vi "controllight.vi"() -> ()   [LabVIEW 2021]
uses:
  <vilib>/Instr/_visa.llb/VISA Configure Serial Port (Instr).vi
panel:
  in  "Reset":bool
  out "TIME":string
  out "Do sang":string
  out "qua toi":bool
  out "qua sang":bool
  out "do sang binh thuong":bool
  out "Waveform Chart":i32(graph)
  in  "write buffer":string
  in  "stop":bool
  out "read buffer":string
  in  "VISA resource name":refnum<visa-resource-name>
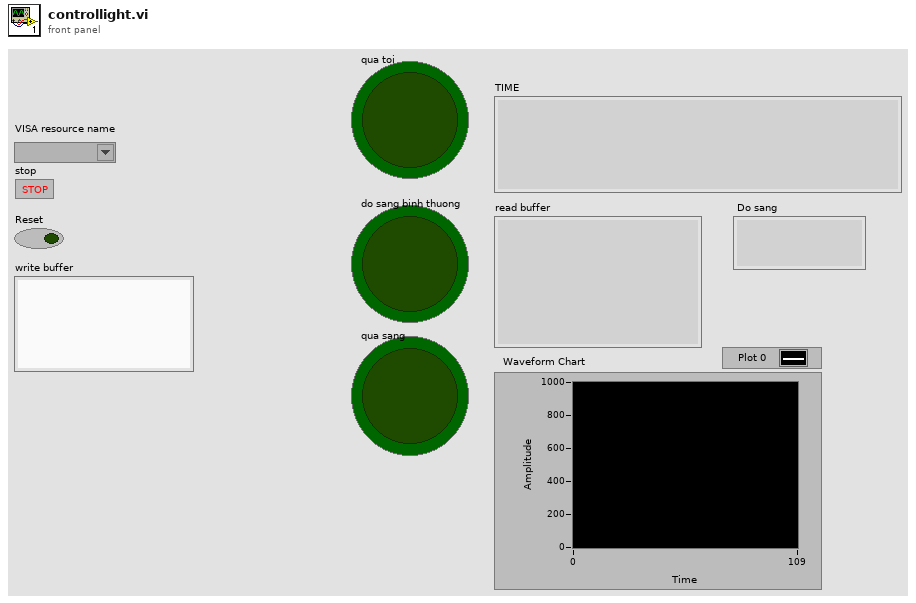
[diagram p1: front panel]
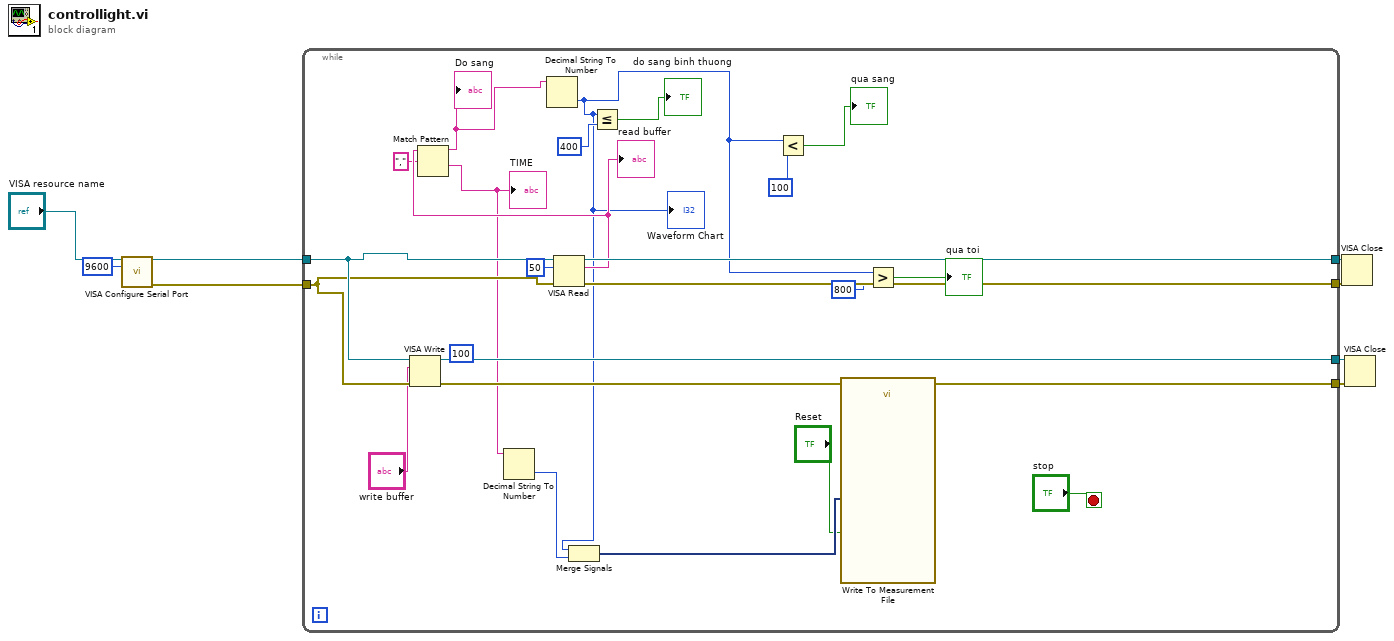
[diagram p0: block diagram]
diagram:
  n1 = call-poly "VISA Configure Serial Port"("VISA resource name"="VISA resource name", "baud rate (9600)"=u32 9600) -> ("VISA resource name out"=w6:refnum<visa-resource-name>, "error out"=w5:errorcluster)  [unwired: 12 in]
  n2 = while {
    tunnel: w6 -> [w27]
    tunnel: w5 -> [w26]
    tunnel: [w30] -> w4
    tunnel: [w29] -> w3
    tunnel: [w25] -> w2
    tunnel: [w24] -> w1
    stop <- "stop" stop-if-true
    (unwired) u32 100 ("byte count")
    n3 = VISA Write(VISA resource name=w27, write buffer="write buffer", error in (no error)=w26) -> (VISA resource name out=w25:refnum<visa-resource-name>, error out=w24:errorcluster)  [unwired: 1 out]
    n4 = VISA Read(VISA resource name=w27, byte count=u32 50, error in (no error)=w26) -> (VISA resource name out=w30:refnum<visa-resource-name>, read buffer=w16:string, error out=w29:errorcluster)  [unwired: 1 out]
    "read buffer" <- w16
    n5 = Match Pattern(string=w16, regular expression=",") -> (before substring=w14:string, after substring=w12:string)  [unwired: 1 in, 2 out]
    "Do sang" <- w14
    "TIME" <- w12
    n6 = Decimal String To Number(string=w12) -> (number=w10:i32)  [unwired: 2 in, 1 out]
    n7 = Decimal String To Number(string=w14) -> (number=w13:i32)  [unwired: 2 in, 1 out]
    "Waveform Chart" <- w13
    n8 = Merge Signals(w13, w10) -> (w11:dynamicdata)
    n9 = Less Or Equal?(x=w13, y=400) -> (x <= y?=→"do sang binh thuong":bool)
    n10 = Less?(x=w13, y=100) -> (x < y?=→"qua sang":bool)
    n11 = call "Write To Measurement File"("Signals"=w11, "Reset"="Reset") -> ()  [unwired: 15 in, 3 out]
    n12 = Greater?(x=w13, y=800) -> (0:→"qua toi":bool)
  }
  n13 = VISA Close(VISA resource name=w4, error in (no error)=w3) -> ()  [unwired: 1 out]
  n14 = VISA Close(VISA resource name=w2, error in (no error)=w1) -> ()  [unwired: 1 out]
